vi "Accelerometer_roll_pitch_student.vi"(11 "Accelerometer Data (x, y, z)":dbl[](array[numeric])) -> (2 "Roll_a":dbl, 3 "Pitch_a":dbl)   [LabVIEW 2014]
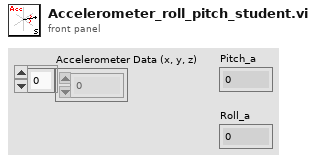
[diagram p1: front panel]
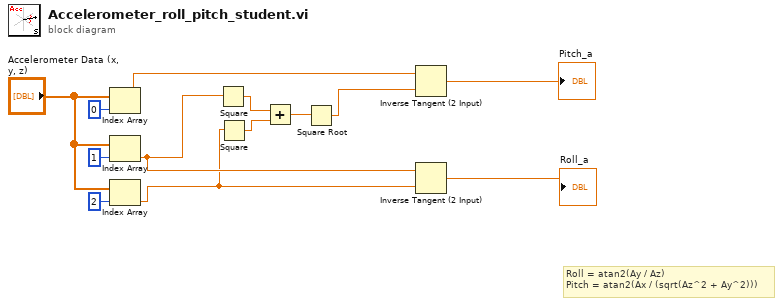
[diagram p0: block diagram]
diagram:
  # "Roll = atan2(Ay / Az)\nPitch = atan2(Ax / (sqrt(Az^2 + Ay^2)))"
  n1 = Index Array(array="Accelerometer Data (x, y, z)", index=0) -> (element=w2:dbl)
  n2 = Index Array(array="Accelerometer Data (x, y, z)", index=1) -> (element=w8:dbl)
  n3 = Index Array(array="Accelerometer Data (x, y, z)", index=2) -> (element=w7:dbl)
  n4 = Square(x=w8) -> (x^2=w6:dbl)
  n5 = Square(x=w7) -> (x^2=w5:dbl)
  n6 = Add(x=w6, y=w5) -> (x+y=w4:dbl)
  n7 = Square Root(x=w4) -> (sqrt(x)=w3:dbl)
  n8 = Inverse Tangent (2 Input)(1:w3, 2:w2) -> (0:→"Pitch_a":dbl)
  n9 = Inverse Tangent (2 Input)(1:w7, 2:w8) -> (0:→"Roll_a":dbl)
